vi "Configure External Sensor Range.vi"(0 "VISA resource name":refnum<visa-resource-name>, 1 "Range Type (1: Custom)":dbl(ring)=1.0 format="%_1g" items=["ALL", "Custom"], 2 "Enable Auto Range (F: Disable)":bool, 5 "Range Configuration (True)":bool[](array[boolean])=[TRUE, TRUE, TRUE, TRUE, TRUE, TRUE, TRUE, TRUE, TRUE], 7 "Enable Peak Over Jump (F: Disable)":bool, 9 "Jump Range (10 <5> V)":dbl(ring)=5.0 items=["50m <25m>"=0.025, "100m <50m>"=0.05, "200m <100m>"=0.1, "500m <250m>"=0.25, "1 <500m>"=0.5, "2 <1>"=1.0, "2.5 <1.25>"=1.25, "5 <2.5m>"=2.5, "10 <5>"=5.0], 11 "error in (no error)":errorcluster, 12 "Manual Range (10 <5> V)":dbl(ring)=5.0 items=["50m <25m>"=0.025, "100m <50m>"=0.05, "200m <100m>"=0.1, "500m <250m>"=0.25, "1 <500m>"=0.5, "2 <1>"=1.0, "2.5 <1.25>"=1.25, "5 <2.5>"=2.5, "10 <5>"=5.0]) -> (4 "VISA resource name out":refnum<visa-resource-name>, 15 "error out":errorcluster)   [LabVIEW 2019, in "Yokogawa WT300 Series.lvlib"]
doc: "Configures the external sensor range features.\n\n<b>Note:</b>\nThis setting valid on models with the external current sensor input (/EX1, /EX2) option."
uses:
  Yokogawa WT300 Series.lvlib
panel:
  # "50m <25m> V"
  # "100m <50m> V"
  # "200m <100m> V"
  # "500m <250m> V"
  # "1 <500m> V"
  # "2 <1> V"
  # "2.5 <1.25> V"
  # "5 <2.5> V"
  # "10 <5> V"
  # "V"
  # "V"
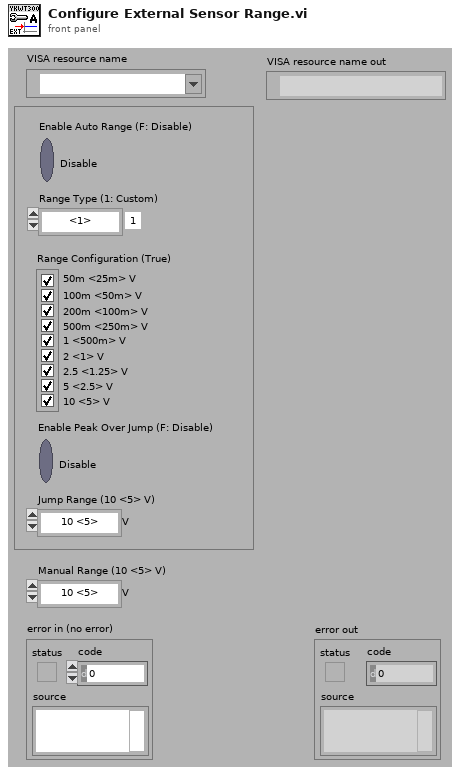
[diagram p1: front panel]
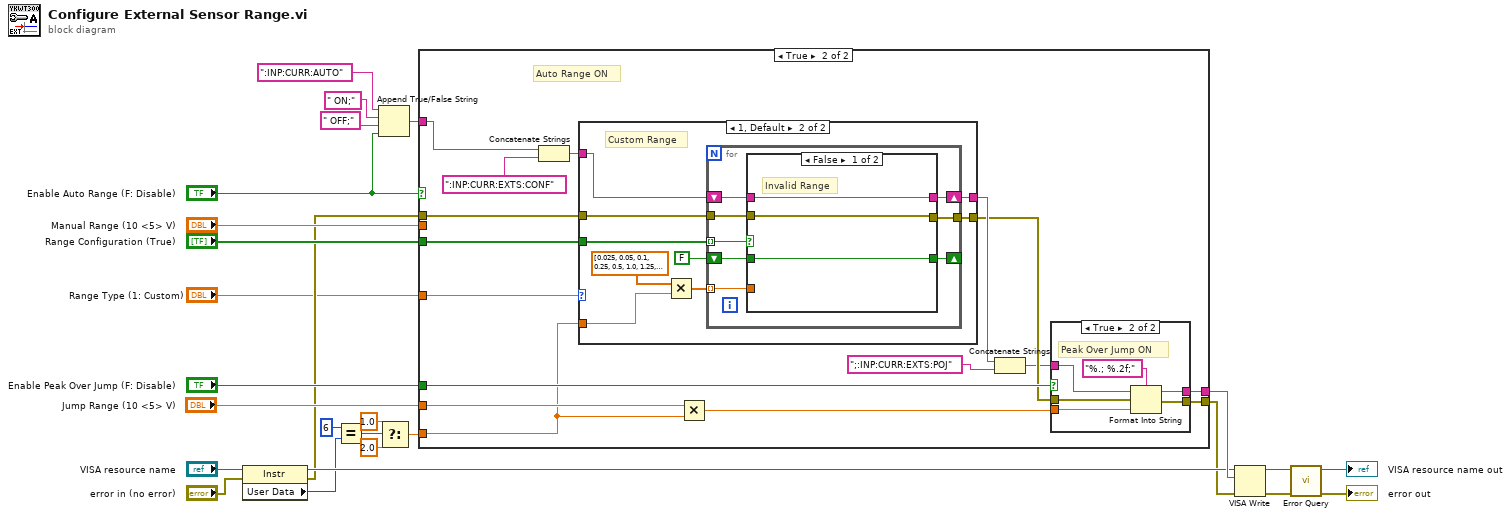
[diagram p0: block diagram]
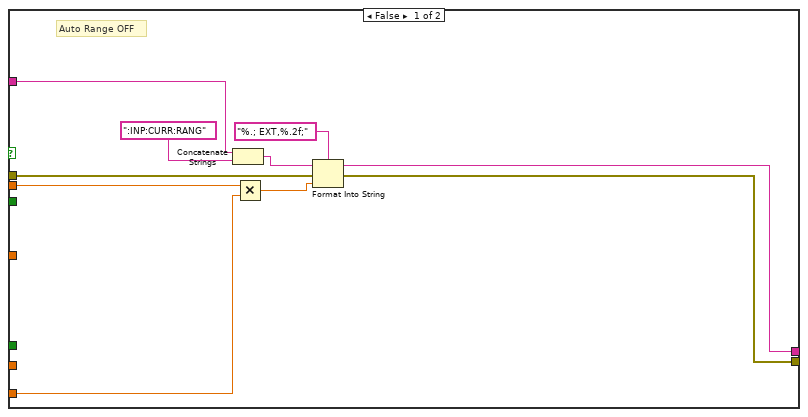
[diagram p2: hidden frame]
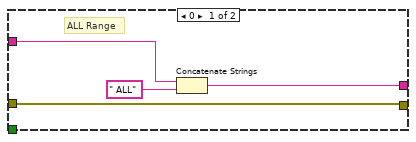
[diagram p3: hidden frame]
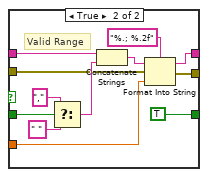
[diagram p4: hidden frame]
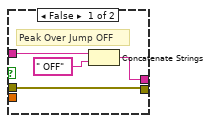
[diagram p5: hidden frame]
diagram:
  n1 = property class="Instr"(reference="VISA resource name", error in="error in (no error)") -> (reference out=w6:refnum<visa-resource-name>, error out=w5:errorcluster, "User Data"=w4:u32)
  n2 = Equal?(x=i64 6 ("y"), y=w4) -> (x = y?=w16:bool)
  n3 = Append True/False String ("True/False 文字列を追加")(1:"Enable Auto Range (F: Disable)", 2:" OFF;", 3:" ON;", 4:":INP:CURR:AUTO") -> (0:w12:string)
  n4 = Select(t=1.0 ("y"), s=w16, f=2.0 ("y")) -> (s? t:f=w14:dbl)
  n5 = case shown="True" "Enable Auto Range (F: Disable)" {
    tunnel: "Manual Range (10 <5> V)" -> [w34 _]
    tunnel: w14 -> [w33 w46]
    tunnel: "Range Configuration (True)" -> [_ w40]
    tunnel: w12 -> [w31 w42]
    tunnel: "Enable Peak Over Jump (F: Disable)" -> [_ w50]
    tunnel: "Jump Range (10 <5> V)" -> [_ w47]
    tunnel: [w30 w49] -> w9
    tunnel: w5 -> [w29 w45]
    tunnel: [w28 w44] -> w1
    tunnel: "Range Type (1: Custom)" -> [_ w39]
    frame False {
      # "Auto Range OFF"
      n6 = Concatenate Strings(w31, ":INP:CURR:RANG") -> (w27:string)
      n7 = Multiply(x=w34, y=w33) -> (x*y=w35:dbl)
      n8 = Format Into String(format string="%.; EXT,%.2f;" ("形式文字列"), initial string=w27, error in=w29, w35) -> (resulting string=w30:string, error out=w28:errorcluster)
    }
    frame True {
      # "Auto Range ON"
      n9 = Concatenate Strings(w42, ":INP:CURR:EXTS:CONF") -> (w52:string)
      n10 = case "ケースストラクチャ" shown="1, Default" w39 {
        tunnel: w52 -> [w56 w58]
        tunnel: [w54 w64] -> w51
        tunnel: w46 -> [_ w57]
        tunnel: w45 -> [w53 w63]
        tunnel: [w53 w62] -> w43
        tunnel: w40 -> [_ w60]
        frame 0 {
          # "ALL Range"
          n11 = Concatenate Strings(w56, " ALL") -> (w54:string)
        }
        frame 1, Default {
          # "Custom Range"
          n12 = Multiply(x=dbl[] [0.025, 0.05, 0.1, 0.25, 0.5, 1.0, 1.25, 2.5, 5.0], y=w57) -> (x*y=w59:dbl[])
          n13 = for {
            tunnel: w60 -> [w71] mode=indexing
            shift-right: [w72] -> w64
            shift-left: w58 -> [w73]
            tunnel: w59 -> [w70] mode=indexing
            tunnel: w63 -> [w69]
            tunnel: [w68] -> w62
            shift-right: [w66] -> _
            shift-left: FALSE -> [w67]
            n14 = case shown="False" w71 {
              tunnel: w73 -> [w76 w86]
              tunnel: [w76 w82] -> w72
              tunnel: w70 -> [_ w81]
              tunnel: w69 -> [w75 w80]
              tunnel: [w75 w79] -> w68
              tunnel: w67 -> [w74 w78]
              tunnel: [w74 TRUE] -> w66
              frame False {
                # "Invalid Range"
              }
              frame True {
                # "Valid Range"
                n15 = Select(t=",", s=w78, f=" ") -> (s? t:f=w85:string)
                n16 = Concatenate Strings(w86, w85) -> (w84:string)
                n17 = Format Into String(format string="%.; %.2f" ("形式文字列"), initial string=w84, error in=w80, w81) -> (resulting string=w82:string, error out=w79:errorcluster)
              }
            }
          }
        }
      }
      n18 = Multiply(x=w47, y=w46) -> (x*y=w48:dbl)
      n19 = Concatenate Strings(w51, ";:INP:CURR:EXTS:POJ") -> (w38:string)
      n20 = case shown="True" w50 {
        tunnel: w38 -> [w91 w97]
        tunnel: w48 -> [_ w96]
        tunnel: [w90 w95] -> w49
        tunnel: [w89 w94] -> w44
        tunnel: w43 -> [w89 w93]
        frame False {
          # "Peak Over Jump OFF"
          n21 = Concatenate Strings(w91, " OFF" ("文字列")) -> (w90:string)
        }
        frame True {
          # "Peak Over Jump ON"
          n22 = Format Into String(format string="%.; %.2f;" ("形式文字列"), initial string=w97, error in=w93, w96) -> (resulting string=w95:string, error out=w94:errorcluster)
        }
      }
    }
  }
  n23 = VISA Write ("VISA書き込み")(VISA resource name=w6, write buffer=w9, error in (no error)=w1) -> (VISA resource name out=w26:refnum<visa-resource-name>, error out=w25:errorcluster)  [unwired: 1 out]
  n24 = call "Error Query.vi"("error in (no error)"=w25, "VISA resource name"=w26) -> ("error out"=→"error out":errorcluster, "VISA resource name out"=→"VISA resource name out":refnum<visa-resource-name>)  [unwired: 6 in, 2 out]
